vi "Assert_Core.vi"(4 "Execution time (s)":dbl=-1.0, 6 "error code (1)":i32=1, 7 "Name":string, 8 "upstream error":errorcluster, 10 "Assert?":bool, 11 "Assert in":refnum<class "Assert.lvclass">) -> (0 "error out":errorcluster, 2 "Properties.Assert":refnum<class "Properties.Assert.lvclass">, 3 "Assert out":refnum<class "Assert.lvclass">)   [LabVIEW 2013, in "Caraya.lvlib" / "Assert.lvclass"]
doc: "Defines how assertion should be handled. Default implementation renders an error if assertion fails."
uses:
  Assert.lvclass
  Properties.Assert/Properties.Assert.lvclass
  Assert.lvclass/Assert.ctl
  Test Assert Factory/Test Assert Factory.lvclass
  Assert Factory Manager/Assert Factory Manager.lvclass
  Caraya.lvlib
  Basic Test Manager/Basic Test Manager.lvclass
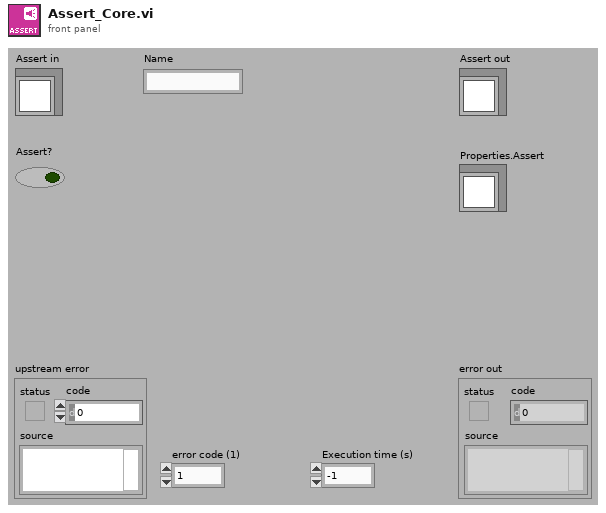
[diagram p1: front panel]
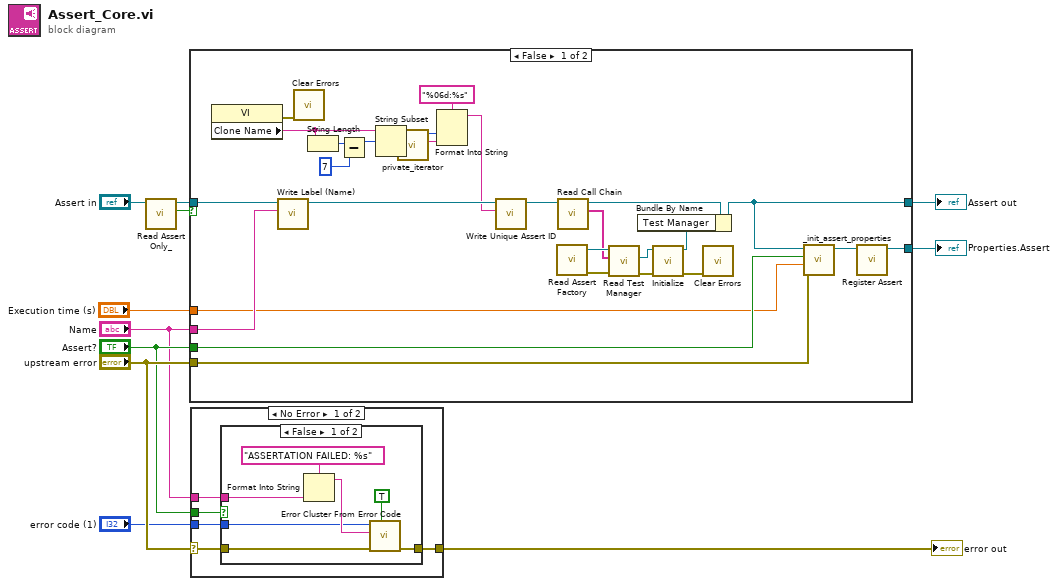
[diagram p0: block diagram]
diagram:
  n1 = call "Read Assert Only_.vi"("Assert"="Assert in") -> ("Assert Only?"=w8:bool, "Assert"=w9:refnum<class "Assert.lvclass">)  [unwired: 8 in, 1 out]
  n2 = case shown="False" w8 {
    tunnel: [w12 w39] -> w6
    tunnel: "Name" -> [w24 _]
    tunnel: "Execution time (s)" -> [w19 _]
    tunnel: "Assert?" -> [w20 _]
    tunnel: "upstream error" -> [w18 _]
    tunnel: w9 -> [w25 w39]
    tunnel: [w21 _] -> w4
    frame False {
      n3 = property class="VI"() -> (error out=w26:errorcluster, "Clone Name"=w27:string)  [unwired: 2 in, 1 out]
      n4 = call "Write Label (Name).vi"("Label"=w24, "Assert in"=w25) -> ("Assert out"=w15:refnum<class "Assert.lvclass">)  [unwired: 9 in]
      n5 = call <vilib>:"Clear Errors.vi"("error in (no error)"=w26) -> ()  [unwired: 6 in, 1 out]
      n6 = String Length(string=w27) -> (length=w33:i32)
      n7 = Subtract(x=w33, y=7) -> (x-y=w35:i32)
      n8 = String Subset(string=w27, offset (0)=w35) -> (substring=w38:string)  [unwired: 1 in]
      n9 = call "private_iterator.vi"() -> ("iterator"=w37:u32)  [unwired: 11 in]
      n10 = Format Into String(format string="%06d:%s", w37, w38) -> (resulting string=w13:string)  [unwired: 2 in, 1 out]
      n11 = call "Write Unique Assert ID.vi"("Unique Assert ID"=w13, "Assert in"=w15) -> ("Assert out"=w14:refnum<class "Assert.lvclass">)  [unwired: 9 in]
      n12 = call "Read Assert Factory.vi"() -> ("error out"=w29:errorcluster, "Test Assert Factory"=w30:refnum<class "Test Assert Factory.lvclass">)  [unwired: 10 in]
      n13 = call "Read Call Chain.vi"("Assert in"=w14) -> ("Call Chain"=w28:string[], "Assert out"=w23:refnum<class "Assert.lvclass">)  [unwired: 9 in]
      n14 = call-dynamic "Read Test Manager.vi"("error in (no error)"=w29, "VI Call Chain"=w28, "Assert Factory in"=w30) -> ("error out"=w31:errorcluster, "Basic Test Manager"=w16:refnum<class "Basic Test Manager.lvclass">)  [unwired: 6 in, 1 out]
      n15 = call "Initialize.vi"("error in (no error)"=w31, "Test Manager in"=w16) -> ("error out"=w32:errorcluster, "Test Manager out"=w22:refnum<class "Basic Test Manager.lvclass">)  [unwired: 8 in]
      n16 = Bundle By Name(cluster=w23, "Test Manager"=w22) -> (w12:refnum<class "Assert.lvclass">)
      n17 = call <vilib>:"Clear Errors.vi"("error in (no error)"=w32) -> ()  [unwired: 6 in, 1 out]
      n18 = call "_init_assert_properties.vi"("upstream error"=w18, "Execution time (s)"=w19, "Asserted"=w20, "Assert in"=w12) -> ("Properties.Assert"=w17:refnum<class "Properties.Assert.lvclass">)  [unwired: 7 in]
      n19 = call "Register Assert.vi"("Properties.Assert in"=w17) -> ("Properties.Assert out"=w21:refnum<class "Properties.Assert.lvclass">)  [unwired: 10 in]
    }
    frame True {
    }
  }
  "Assert out" <- w6
  "Properties.Assert" <- w4
  n20 = case shown="No Error" "upstream error" {
    selector: "upstream error" -> [w44 w53]
    tunnel: [w43 w53] -> w7
    tunnel: "Assert?" -> [w40 _]
    tunnel: "Name" -> [w42 _]
    tunnel: "error code (1)" -> [w41 _]
    frame No Error {
      n21 = case shown="False" w40 {
        tunnel: w44 -> [w48 w52]
        tunnel: [w51 w52] -> w43
        tunnel: w42 -> [w49 _]
        tunnel: w41 -> [w45 _]
        frame False {
          n22 = Format Into String(format string="ASSERTATION FAILED: %s", w49) -> (resulting string=w47:string)  [unwired: 2 in, 1 out]
          n23 = call <vilib>:"Error Cluster From Error Code.vi"("show call chain? (False)"=TRUE, "error in (no error)"=w48, "error message (\"\")"=w47, "error code (0)"=w45) -> ("error out"=w51:errorcluster)  [unwired: 5 in]
        }
        frame True {
        }
      }
    }
    frame Error {
    }
  }
  "error out" <- w7
